vi "GetPlayer1Position.vi"(8 "error in (no error)":errorcluster, 11 "Board in":refnum<class "Board.lvclass">) -> (0 "error out":errorcluster, 2 "Player1Position":T1, 3 "Board out":refnum<class "Board.lvclass">)   [LabVIEW 2015, in "TronviewGame.lvlib" / "Board.lvclass"]
uses:
  Board.lvclass
  Position.ctl
  Board.lvclass/Board.ctl
  FieldState.ctl
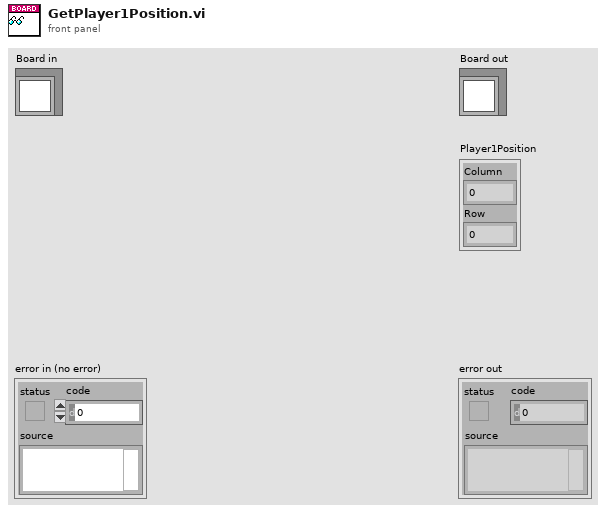
[diagram p1: front panel]
types:
  T1 = typedef "TronviewGame.lvlib/Board.lvclass/Position.ctl" = cluster{"Column":i32, "Row":i32}
  T2 = typedef "TronviewGame.lvlib/Board.lvclass/FieldState.ctl" = enum16{"Empty", "Blocked", "Player1Position", "Player2Postion", "Player1Marked", "Player2Marked"}
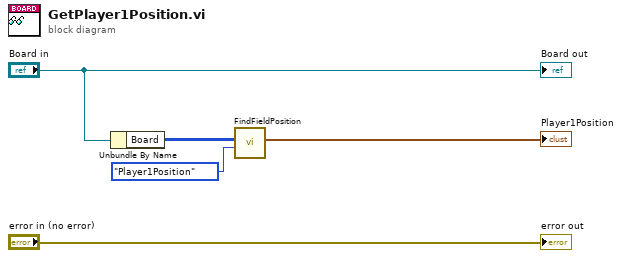
[diagram p0: block diagram]
diagram:
  n1 = Unbundle By Name("Board in") -> ("Board"=w3:T2[][])
  n2 = call "FindFieldPosition.vi"("Field"=FieldState."Player1Position", "Board"=w3) -> ("Position"=→"Player1Position":T1)  [unwired: 8 in, 1 out]
  "error out" <- "error in (no error)"
  "Board out" <- "Board in"
